vi "sub_camerafile_update.vi"(11 "camera_attrib":cluster{"brightness":u16, "ExposureTimeAbs":dbl} {"brightness" scale=0.0..10.0; "ExposureTimeAbs" scale=0.0..10.0}) -> ()   [LabVIEW 2019]
uses:
  <vilib>/vision/driver/NI_Vision_Acquisition_Software.lvlib
panel:
  in  "error out":errorcluster
  in  "error in":errorcluster
  out "camera file data":string
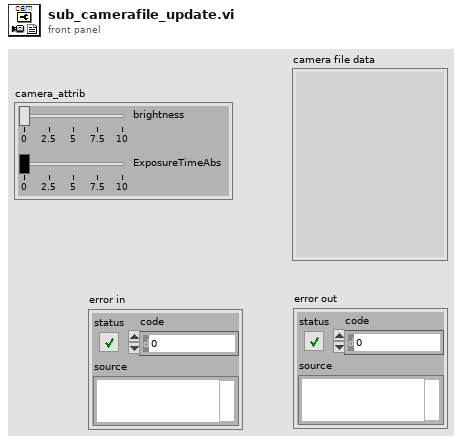
[diagram p1: front panel]
types:
  T1 = enum16{"open", "replace", "create", "open or create", "replace or create", "replace or create with confirmation"}
  T2 = typedef "IMAQdx.ctl" = refnum<k21>
  T3 = typedef "IMAQ Image.ctl" = refnum<image>
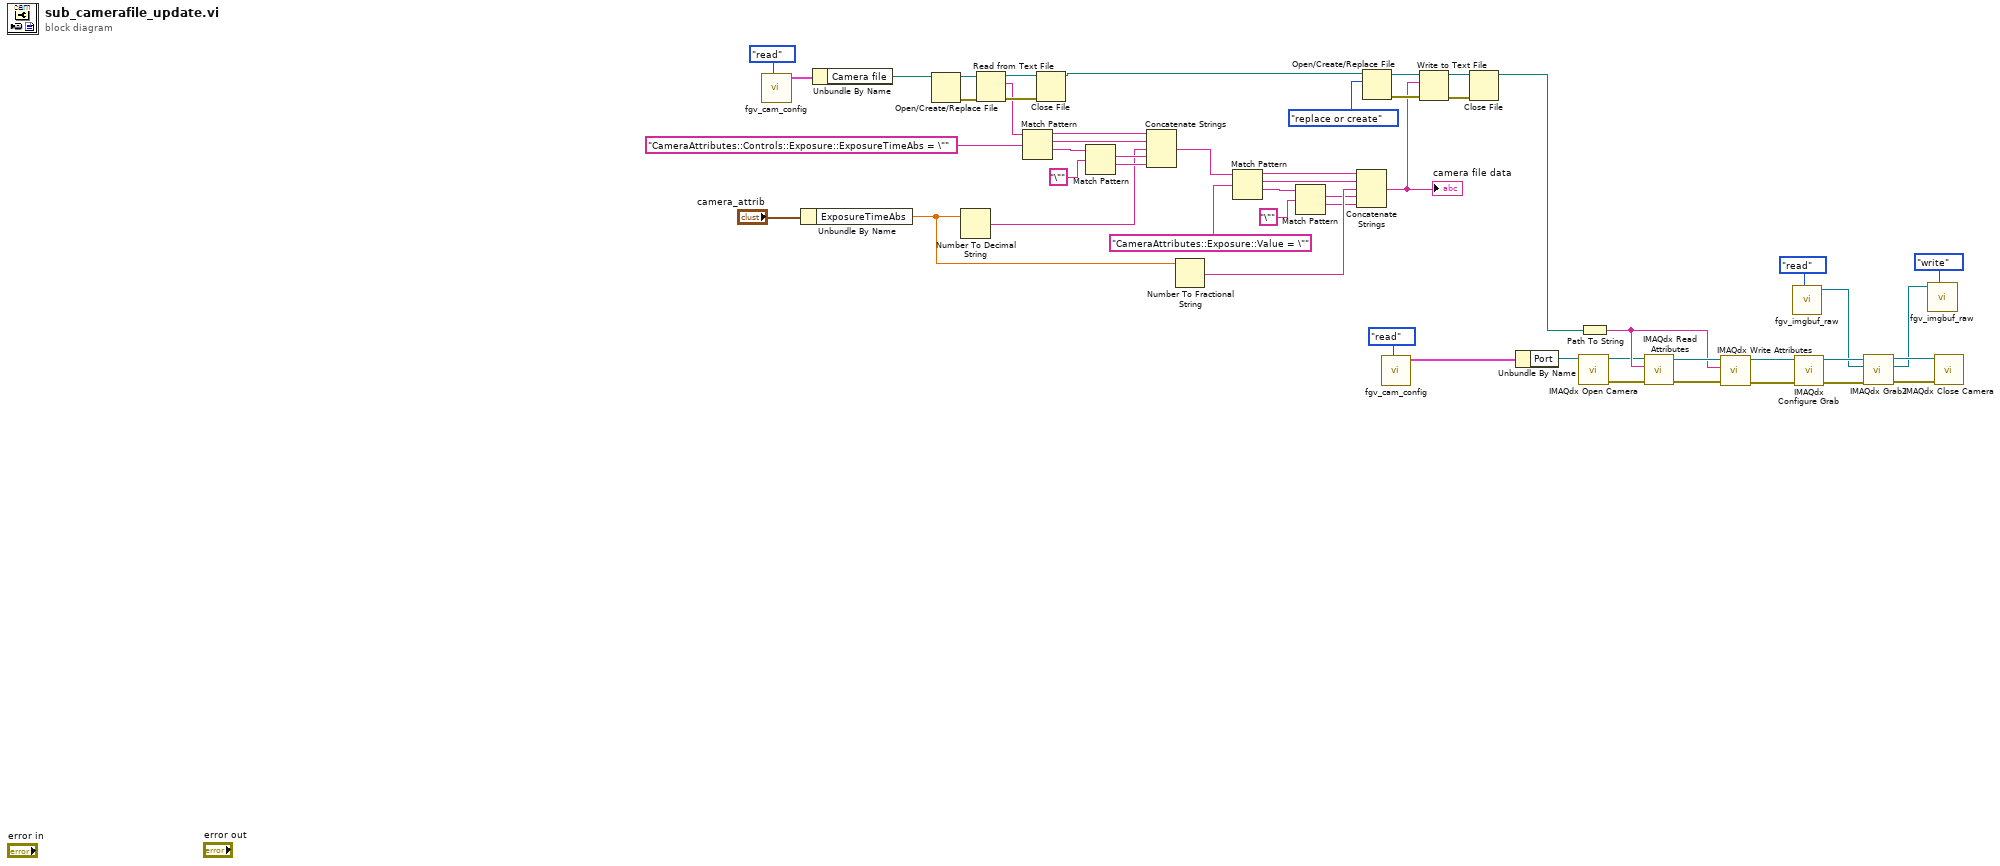
[diagram p0: block diagram]
diagram:
  n1 = call "fgv_cam_config.vi"("cmd"=enum16{"read", "write"}."read") -> ("camera cfg out"=w18:cluster{"Port":T2, "Camera file":path})  [unwired: 10 in]
  n2 = Unbundle By Name("camera_attrib") -> ("ExposureTimeAbs"=w16:dbl)
  n3 = Unbundle By Name(w18) -> ("Camera file"=w17:path)
  n4 = Open/Create/Replace File(file path (use dialog)=w17) -> (refnum out=w48:refnum<file>, error out=w47:errorcluster)  [unwired: 5 in, 1 out]
  n5 = Number To Decimal String(number=w16) -> (decimal integer string=w26:string)  [unwired: 1 in]
  n6 = Read from Text File(file (use dialog)=w48, error in=w47) -> (refnum out=w51:refnum<file>, text=w49:string, error out=w50:errorcluster)  [unwired: 2 in, 1 out]
  n7 = Match Pattern(string=w49, regular expression="CameraAttributes::Controls::Exposure::ExposureTimeAbs = \"") -> (before substring=w25:string, match substring=w28:string, after substring=w23:string)  [unwired: 1 in, 1 out]
  n8 = Close File(refnum=w51, error in=w50) -> (path=w52:path)  [unwired: 1 out]
  n9 = Match Pattern(string=w23, regular expression="\"") -> (match substring=w29:string, after substring=w27:string)  [unwired: 1 in, 2 out]
  n10 = Concatenate Strings(w25, w28, w26, w29, w27) -> (w53:string)
  n11 = Number To Fractional String(number=w16) -> (F-format string=w37:string)  [unwired: 3 in]
  n12 = Match Pattern(string=w53, regular expression="CameraAttributes::Exposure::Value = \"") -> (before substring=w33:string, match substring=w31:string, after substring=w35:string)  [unwired: 1 in, 1 out]
  n13 = Match Pattern(string=w35, regular expression="\"") -> (match substring=w30:string, after substring=w32:string)  [unwired: 1 in, 2 out]
  n14 = Concatenate Strings(w33, w31, w37, w30, w32) -> (w20:string)
  "camera file data" <- w20
  n15 = Open/Create/Replace File(file path (use dialog)=w52, operation (0:open)=T1."replace or create") -> (refnum out=w42:refnum<file>, error out=w39:errorcluster)  [unwired: 4 in, 1 out]
  n16 = call "fgv_cam_config.vi"("cmd"=enum16{"read", "write"}."read") -> ("camera cfg out"=w8:cluster{"Port":T2, "Camera file":path})  [unwired: 10 in]
  n17 = Write to Text File(file (use dialog)=w42, text=w20, error in=w39) -> (refnum out=w41:refnum<file>, error out=w40:errorcluster)  [unwired: 1 in, 1 out]
  n18 = Close File(refnum=w41, error in=w40) -> (path=w44:path)  [unwired: 1 out]
  n19 = Unbundle By Name(w8) -> ("Port"=w7:T2)
  n20 = call <vilib>:"IMAQdx Open Camera.vi"("Session In"=w7) -> ("error out"=w5:errorcluster, "Session Out"=w6:T2)  [unwired: 9 in]
  n21 = Path To String(path=w44) -> (string=w21:string)
  n22 = call <vilib>:"IMAQdx Read Attributes.vi"("error in"=w5, "Filename"=w21, "Session In"=w6) -> ("error out"=w45:errorcluster, "Session Out"=w46:T2)  [unwired: 7 in]
  n23 = call <vilib>:"IMAQdx Write Attributes.vi"("error in"=w45, "Filename"=w21, "Session In"=w46) -> ("error out"=w13:errorcluster, "Session Out"=w12:T2)  [unwired: 7 in]
  n24 = call "fgv_imgbuf_raw.vi"("cmd"=enum16{"create", "close", "write", "read"}."read") -> ("Image"=w3:T3)  [unwired: 9 in, 1 out]
  n25 = call <vilib>:"IMAQdx Configure Grab.vi"("error in"=w13, "Session In"=w12) -> ("error out"=w15:errorcluster, "Session Out"=w14:T2)  [unwired: 8 in]
  n26 = call <vilib>:"IMAQdx Grab2.vi"("error in"=w15, "Image In"=w3, "Session In"=w14) -> ("error out"=w10:errorcluster, "Image Out"=w1:T3, "Session Out"=w11:T2)  [unwired: 5 in, 1 out]
  n27 = call "fgv_imgbuf_raw.vi"("cmd"=enum16{"create", "close", "write", "read"}."write", "raw Image in"=w1) -> ()  [unwired: 8 in, 2 out]
  n28 = call <vilib>:"IMAQdx Close Camera.vi"("error in"=w10, "Session In"=w11) -> ()  [unwired: 9 in, 1 out]
